vi "Correct_Position_info_NM.vi"() -> (0 "error out":errorcluster, 4 "Path":path)   [LabVIEW 2015]
panel:
  out "Array":path[](array[path])
  out "File Changed":bool
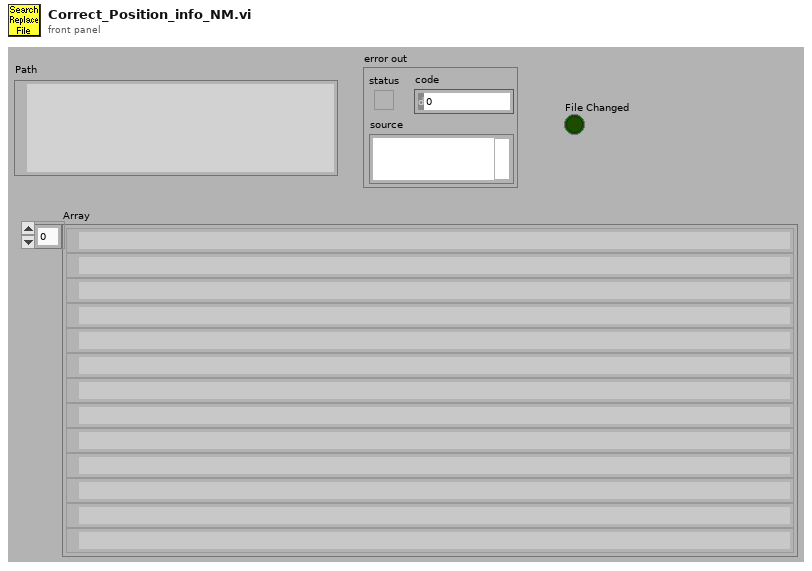
[diagram p1: front panel]
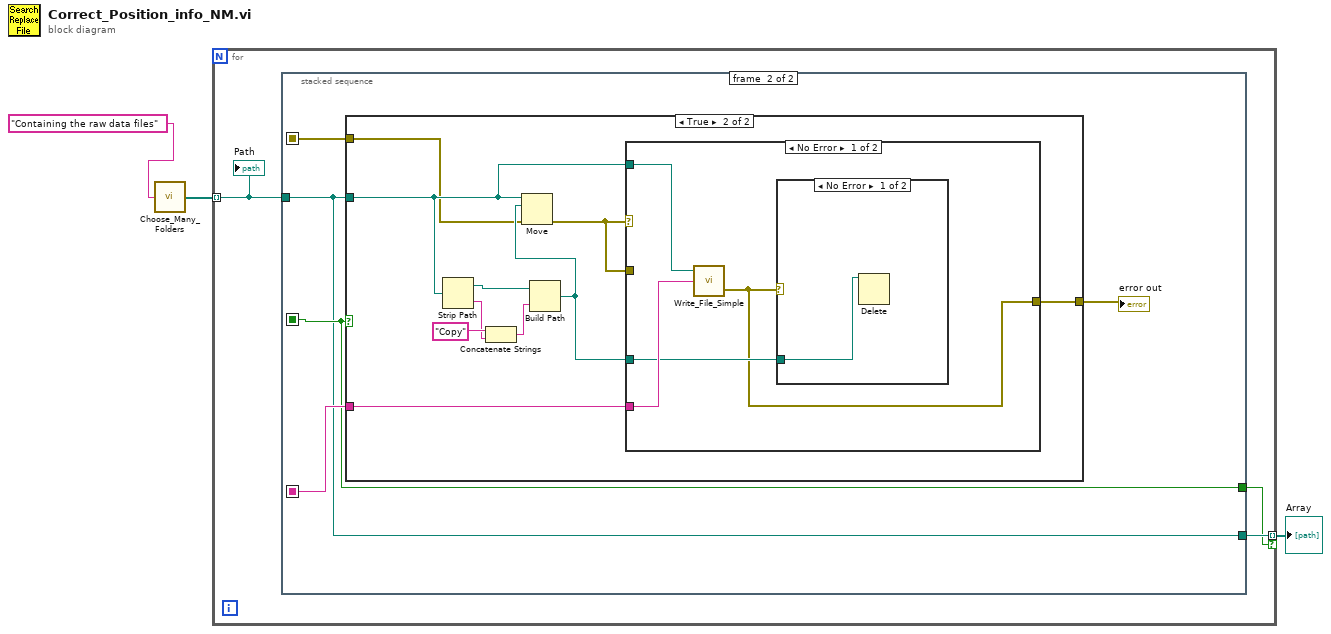
[diagram p0: block diagram]
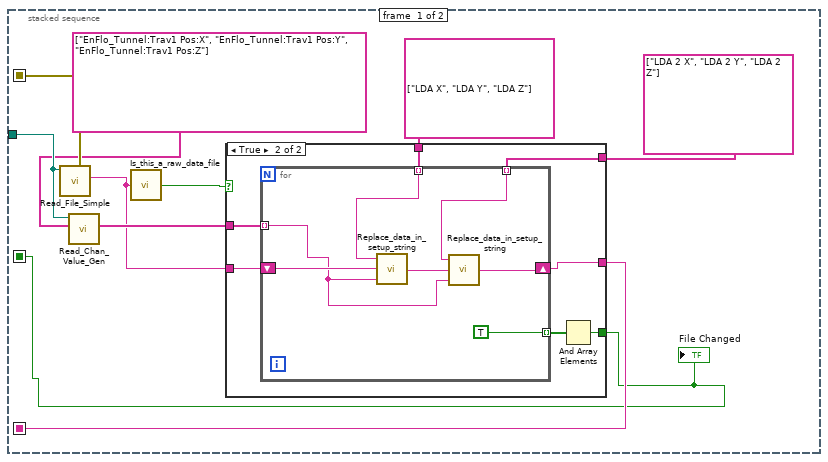
[diagram p2: hidden frame]
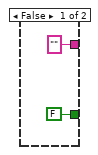
[diagram p3: hidden frame]
diagram:
  n1 = call "Choose_Many_Folders.vi"("Purpose of choosing folder"="Containing the raw data files") -> ("Files"=w2:path[])
  n2 = for {
    tunnel: w2 -> [w6] mode=indexing
    tunnel: [w5] -> w1 mode=indexing if=w4
    n3 = stacked-sequence {
      seq-local: [w16 _] -> [_ w36]
      seq-local: [w14 _] -> [_ w35]
      seq-local: [w12 _] -> [_ w34]
      tunnel: w6 -> [w11 w33]
      tunnel: [_ w33] -> w5
      tunnel: [_ w34] -> w4
      frame #0 {
        n4 = call "Read_File_Simple.vi"("Filename"=w11) -> ("error out"=w16:errorcluster, "string"=w8:string)  [unwired: 4 in, 4 out]
        n5 = call "Read_Chan_Value_Gen.vi"("Desired Ch Names"=string[] ["EnFlo_Tunnel:Trav1 Pos:X", "EnFlo_Tunnel:Trav1 Pos:Y", "EnFlo_Tunnel:Trav1 Pos:Z"], "Raw data file"=w11) -> ("Values"=w10:string[])  [unwired: 9 in]
        n6 = call "Is_this_a_raw_data_file.vi"("character string"=w8) -> ("Raw Dat File?"=w7:bool)  [unwired: 2 out]
        n7 = case shown="True" w7 {
          tunnel: string[] ["LDA X", "LDA Y", "LDA Z"] -> [_ w25]
          tunnel: ["" ("string") w24] -> w14
          tunnel: string[] ["LDA 2 X", "LDA 2 Y", "LDA 2 Z"] -> [_ w23]
          tunnel: [FALSE w21] -> w12
          tunnel: w10 -> [_ w20]
          tunnel: w8 -> [_ w19]
          frame False {
          }
          frame True {
            n8 = for {
              shift-right: [w29] -> w24
              shift-left: w19 -> [w30]
              tunnel: w25 -> [w32] mode=indexing
              tunnel: w23 -> [w31] mode=indexing
              tunnel: [TRUE] -> w22 mode=indexing
              tunnel: w20 -> [w27] mode=indexing
              n9 = call "Replace_data_in_setup_string.vi"("New data string"=w27, "Input string"=w30, "Variable name"=w32) -> ("Appended string"=w26:string)
              n10 = call "Replace_data_in_setup_string.vi"("New data string"=w27, "Input string"=w26, "Variable name"=w31) -> ("Appended string"=w29:string)
            }
            n11 = And Array Elements(Boolean array=w22) -> (logical AND=w21:bool)
          }
        }
        "File Changed" <- w12
      }
      frame #1 {
        n12 = case shown="True" w34 {
          tunnel: w33 -> [_ w44]
          tunnel: w35 -> [_ w43]
          tunnel: [w38 w41] -> w37
          tunnel: w36 -> [w38 w39]
          frame False {
          }
          frame True {
            n13 = Strip Path(path=w44) -> (stripped path=w45:path, name=w47:string)
            n14 = Concatenate Strings("Copy" ("name or relative path"), w47) -> (w46:string)
            n15 = Build Path(base path=w45, name or relative path=w46) -> (appended path=w42:path)
            n16 = Move(source path=w44, error in=w39, 10:w42) -> (error out=w40:errorcluster)  [unwired: 2 in, 2 out]
            n17 = case shown="No Error" w40 {
              tunnel: w44 -> [w52 _]
              tunnel: w43 -> [w51 _]
              tunnel: w42 -> [w50 _]
              tunnel: [w49 w54] -> w41
              tunnel: w40 -> [_ w54]
              frame No Error {
                n18 = call "Write_File_Simple.vi"("character string"=w51, "file path"=w52) -> ("error out"=w49:errorcluster)  [unwired: 1 in, 1 out]
                n19 = case shown="No Error" w49 {
                  tunnel: w50 -> [w53 _]
                  frame No Error {
                    n20 = Delete(path (use dialog)=w53) -> ()  [unwired: 4 in, 3 out]
                  }
                  frame Error {
                  }
                }
              }
              frame Error {
              }
            }
          }
        }
        "error out" <- w37
      }
    }
    "Path" <- w6
  }
  "Array" <- w1
